vi "KeyDown Response.vi"(6 "PlatMods":T2, 8 "error in (no error)":errorcluster, 9 "VKey":T1, 10 "Char":i16, 11 "Editor Handler in":refnum<class "Image Editor Handler.lvclass">) -> (0 "error out":errorcluster, 3 "Editor Handler out":refnum<class "Image Editor Handler.lvclass">)   [LabVIEW 2017, in "LV Image Editor Framework.lvlib" / "Image Editor Handler.lvclass"]
uses:
  <vilib>/LIEF/Image Editor Handler/Image Editor Handler.lvclass
  <vilib>/event_ctls.llb/eventvkey.ctl
  <vilib>/Utility/miscctls.llb/LVPoint32TypeDef.ctl
  <vilib>/LIEF/Image Editor Handler/Image Editor Handler.lvclass/Image Editor Handler.ctl
  <vilib>/LIEF/Forms/Selection/Selection.lvclass
  <vilib>/LIEF/Forms/Shape/Shape.lvclass/Shape.ctl
  <vilib>/LIEF/Forms/Shape/Read Selectable.vi
  <vilib>/LIEF/Forms/Shape/Shape.lvclass
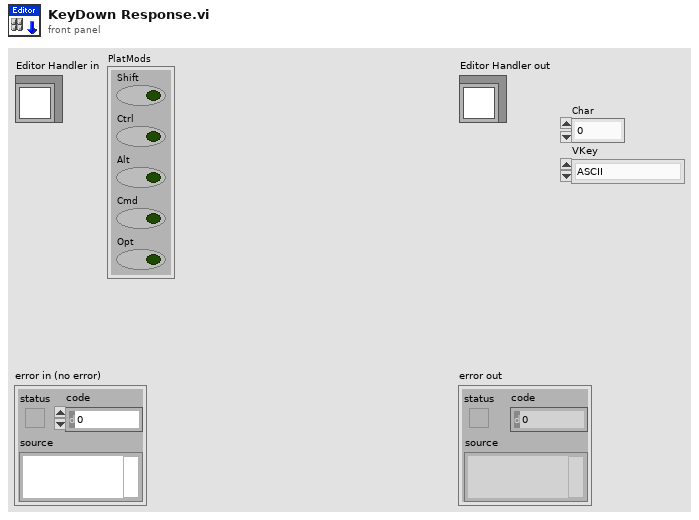
[diagram p1: front panel]
types:
  T1 = typedef "eventvkey.ctl" = enum16{"ASCII", "Enter", "Return", "Shift", "Ctrl", "Alt", "Cmd", "Opt", "Caps", "NumLock", "Clear", "Break", "Up", "Down", "Left", "Right", "Insert", "Delete", "Home", "End", "PageUp", "PageDown", "Escape", "Help", "Pause", "ScrollLock", "F1", "F2", "F3", "F4", "F5", "F6", "F7", "F8", "F9", "F10", "F11", "F12", "F13", "F14", "F15", "F16", "F17", "F18", "F19", "F20", "F21", "F22", "F23", "F24", "Play", "VolumeUp", "VolumeDown", "Mute", "Two Byte Char"}
  T2 = cluster{"Shift":bool, "Ctrl":bool, "Alt":bool, "Cmd":bool, "Opt":bool}
  T3 = typedef "LVPoint32TypeDef.ctl" = cluster{"Horizontal":i32, "Vertical":i32}
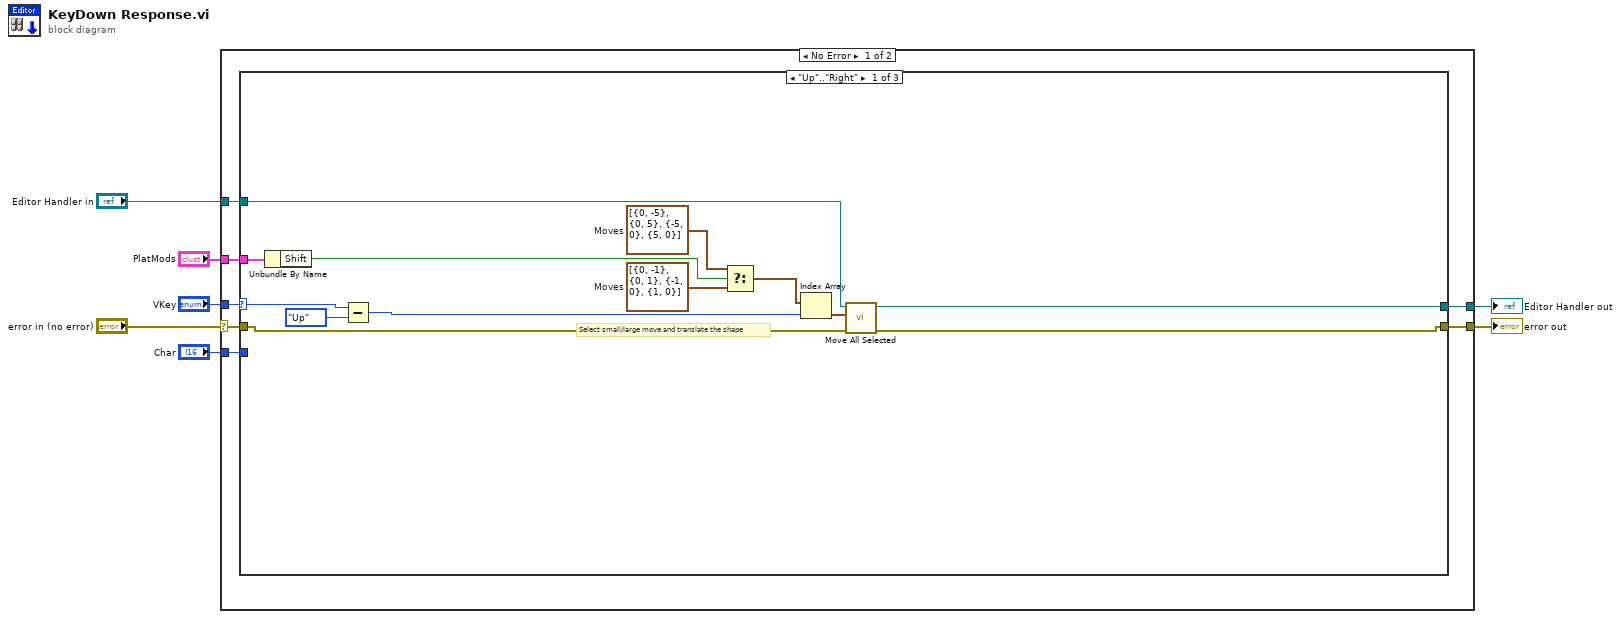
[diagram p0: block diagram]
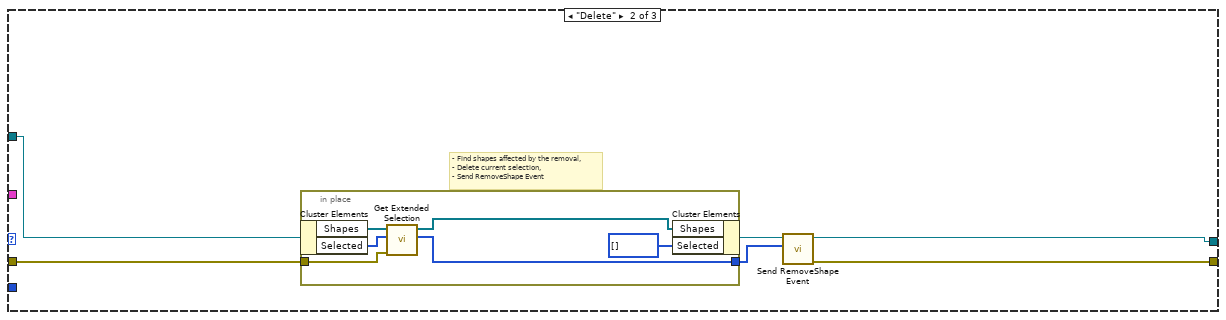
[diagram p2: hidden frame]
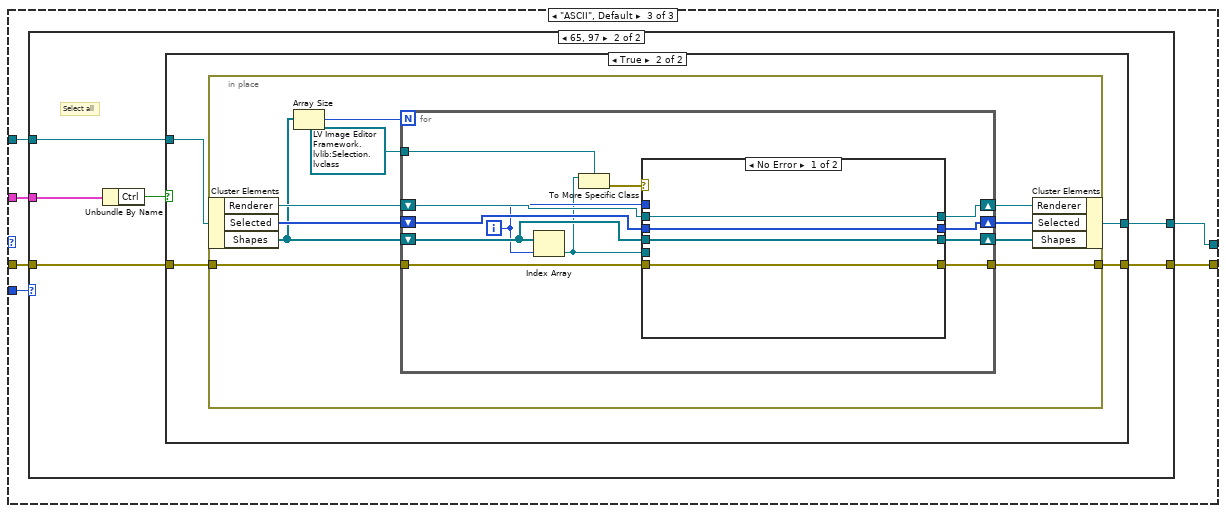
[diagram p3: hidden frame]
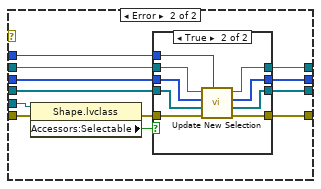
[diagram p6: hidden frame]
diagram:
  n1 = case shown="No Error" "error in (no error)" {
    selector: "error in (no error)" -> [w11 w112]
    tunnel: [w10 w112] -> w3
    tunnel: [w12 w111] -> w1
    tunnel: "Editor Handler in" -> [w14 w111]
    tunnel: "VKey" -> [w13 _]
    tunnel: "PlatMods" -> [w9 _]
    tunnel: "Char" -> [w8 _]
    frame No Error {
      n2 = case shown="\"Up\"..\"Right\"" w13 {
        selector: w13 -> [w20 _ _]
        tunnel: w14 -> [w18 w33 w45]
        tunnel: [w17 w31 w40] -> w12
        tunnel: w11 -> [w15 w29 w42]
        tunnel: [w16 w28 w41] -> w10
        tunnel: w9 -> [w27 _ w44]
        tunnel: w8 -> [_ _ w43]
        frame "Up".."Right" {
          w25 = T3[] [{"Horizontal"=0, "Vertical"=-5}, {"Horizontal"=0, "Vertical"=5}, {"Horizontal"=-5, "Vertical"=0}, {"Horizontal"=5, "Vertical"=0}]  # Moves
          w24 = T3[] [{"Horizontal"=0, "Vertical"=-1}, {"Horizontal"=0, "Vertical"=1}, {"Horizontal"=-1, "Vertical"=0}, {"Horizontal"=1, "Vertical"=0}]  # Moves
          # "Select small/large move and translate the shape"
          n3 = Unbundle By Name(w27) -> ("Shift"=w26:bool)
          n4 = Subtract(x=w20, y=eventvkey."Up") -> (x-y=w23:u16)
          n5 = Select(t=w25, s=w26, f=w24) -> (s? t:f=w21:T3[])
          n6 = Index Array(array=w21, index=w23) -> (element=w19:T3)
          n7 = call <vilib>:"Move All Selected.vi"("error in (no error)"=w15, "Delta"=w19, "Editor Handler in"=w18) -> ("error out"=w16:errorcluster, "Editor Handler out"=w17:refnum<class "Image Editor Handler.lvclass">)  [unwired: 7 in]
        }
        frame "Delete" {
          # "- Find shapes affected by the removal,\n- Delete current selection,\n- Send RemoveShape Event"
          n8 = in-place {
            in-place-border: [w36] -> w30
            in-place-border: w29 -> [w35]
            n9 = in-place-cluster #1(w33) -> ("Shapes"=w37:refnum<data-value>[], "Selected"=w38:i16[])
            n10 = call <vilib>:"Get Extended Selection.vi"("error in (no error)"=w35, "Selected"=w38, "Shapes"=w37) -> ("Ext. Selection"=w36:i32[], "Shapes out"=w34:refnum<data-value>[])  [unwired: 6 in, 1 out]
            n11 = in-place-cluster #1("Shapes"=w34, "Selected"=i16[] []) -> (w32:refnum<class "Image Editor Handler.lvclass">)
          }
          n12 = call <vilib>:"Send RemoveShape Event.vi"("Indexes"=w30, "Editor Handler in"=w32) -> ("error out"=w28:errorcluster, "Editor Handler out"=w31:refnum<class "Image Editor Handler.lvclass">)  [unwired: 8 in]
        }
        frame "ASCII", Default {
          n13 = case shown="65, 97" w43 {
            tunnel: w44 -> [_ w53]
            tunnel: [w46 w52] -> w40
            tunnel: w42 -> [w47 w51]
            tunnel: [w47 w50] -> w41
            tunnel: w45 -> [w46 w49]
            frame Default {
            }
            frame 65, 97 {
              # "Select all"
              n14 = Unbundle By Name(w53) -> ("Ctrl"=w48:bool)
              n15 = case shown="True" w48 {
                tunnel: w49 -> [w55 w59]
                tunnel: [w55 w58] -> w52
                tunnel: w51 -> [w54 w57]
                tunnel: [w54 w56] -> w50
                frame False {
                }
                frame True {
                  n16 = in-place {
                    in-place-border: w57 -> [w66]
                    in-place-border: [w65] -> w56
                    n17 = in-place-cluster #2(w59) -> ("Renderer"=w68:refnum<class "Image.lvclass">, "Selected"=w69:i16[], "Shapes"=w61:refnum<data-value>[])
                    n18 = Array Size(array=w61) -> (size(s)=w60:i32)
                    n19 = for {
                      N: w60 -> [_]
                      shift-right: [w75] -> w64
                      shift-left: w68 -> [w80]
                      shift-right: [w76] -> w63
                      shift-left: w69 -> [w81]
                      shift-right: [w74] -> w62
                      shift-left: w61 -> [w79]
                      tunnel: refnum<data-value> refnum ("target class") -> [w78]
                      tunnel: w66 -> [w73]
                      tunnel: [w72] -> w65
                      i -> [w71]
                      n20 = Index Array(array=w79, index=w71) -> (element=w70:refnum<data-value>)
                      n21 = To More Specific Class(target class=w78, reference=w70) -> (error out=w77:errorcluster)  [unwired: 1 in, 1 out]
                      n22 = case shown="No Error" w77 {
                        tunnel: w81 -> [w85 w97]
                        tunnel: w80 -> [w84 w96]
                        tunnel: w79 -> [w83 w95]
                        tunnel: [w85 w92] -> w76
                        tunnel: [w84 w93] -> w75
                        tunnel: [w83 w91] -> w74
                        tunnel: w73 -> [w82 w90]
                        tunnel: [w82 w88] -> w72
                        tunnel: w71 -> [_ w87]
                        tunnel: w70 -> [_ w86]
                        frame No Error {
                        }
                        frame Error {
                          n23 = property class="Shape.lvclass"(reference=w86, error in=w90) -> (error out=w89:errorcluster, "Accessors:Selectable"=w94:bool)  [unwired: 1 out]
                          n24 = case shown="True" w94 {
                            tunnel: w97 -> [w99 w110]
                            tunnel: w96 -> [w98 w109]
                            tunnel: w95 -> [w100 w108]
                            tunnel: [w98 w107] -> w93
                            tunnel: [w99 w106] -> w92
                            tunnel: [w100 w105] -> w91
                            tunnel: w89 -> [w101 w104]
                            tunnel: [w101 w103] -> w88
                            tunnel: w87 -> [_ w102]
                            frame False {
                            }
                            frame True {
                              n25 = call <vilib>:"Update New Selection.vi"("Node ID"=w102, "error in (no error)"=w104, "Shape in"=w108, "Selected in"=w110, "Image in"=w109) -> ("error out"=w103:errorcluster, "Shape out 2"=w105:refnum<data-value>[], "Selected out 2"=w106:i16[], "Image out"=w107:refnum<class "Image.lvclass">)  [unwired: 3 in]
                            }
                          }
                        }
                      }
                    }
                    n26 = in-place-cluster #2("Renderer"=w64, "Selected"=w63, "Shapes"=w62) -> (w58:refnum<class "Image Editor Handler.lvclass">)
                  }
                }
              }
            }
          }
        }
      }
    }
    frame Error {
    }
  }
  "error out" <- w3
  "Editor Handler out" <- w1
